vi "Find Color.vi"(8 "error in (no error)":errorcluster, 10 "Color Selected":u32(colorbox), 11 "ColorSelector in":refnum<class "ColorSelector.lvclass">) -> (0 "error out":errorcluster, 3 "ColorSelector out":refnum<class "ColorSelector.lvclass">)   [LabVIEW 2015, in "ColorSelector.lvclass"]
doc: "This VI finds the closest color in the Color Selector.\n<b> </b> <b> </b>\n©2017 Q Software Innovations, LLC (QSI)\nwritten by Quentin Alldredge\nproduced in LabVIEW 2015\n\nsupport@qsoftwareinnovations.com\nwww.qsoftwareinnovations.com\n\nAll rights reserved.\n\nRedistribution and use in source and binary forms, with or without modification, are permitted provided that the following conditions are met:\n\n * Redistributions of source code must retain the above copyright notice, this list of conditions and the following disclaimer.\n * Redistributions in binary form must reproduce the above copyright notice, this list of conditions and the following disclaimer in the documentation and/or other materials provided with the distribution.\n * Neither the name of Q Software Innovations, LLC. nor the names of its contributors may be used to endorse or promote products derived from this software without specific prior written permission.\n\nTHIS SOFTWARE IS PROVIDED BY THE COPYRIGHT HOLDERS AND CONTRIBUTORS \"AS IS\" AND ANY EXPRESS OR IMPLIED WARRANTIES, INCLUDING, BUT NOT LIMITED TO, THE IMPLIED WARRANTIES OF MERCHANTABILITY AND FITNESS FOR A PARTICULAR PURPOSE ARE DISCLAIMED. IN NO EVENT SHALL THE COPYRIGHT OWNER OR CONTRIBUTORS BE LIABLE FOR ANY DIRECT, INDIRECT, INCIDENTAL, SPECIAL, EXEMPLARY, OR CONSEQUENTIAL DAMAGES (INCLUDING, BUT NOT LIMITED TO, PROCUREMENT OF SUBSTITUTE GOODS OR SERVICES; LOSS OF USE, DATA, OR PROFITS; OR BUSINESS INTERRUPTION) HOWEVER CAUSED AND ON ANY THEORY OF LIABILITY, WHETHER IN CONTRACT, STRICT LIABILITY, OR TORT (INCLUDING NEGLIGENCE OR OTHERWISE) ARISING IN ANY WAY OUT OF THE USE OF THIS SOFTWARE, EVEN IF ADVISED OF THE POSSIBILITY OF SUCH DAMAGE."
uses:
  ColorSelector.lvclass
  <vilib>/Utility/miscctls.llb/LVPoint32TypeDef.ctl
  Read ColorSelectPic.vi
  Write ColorGridCoords.vi
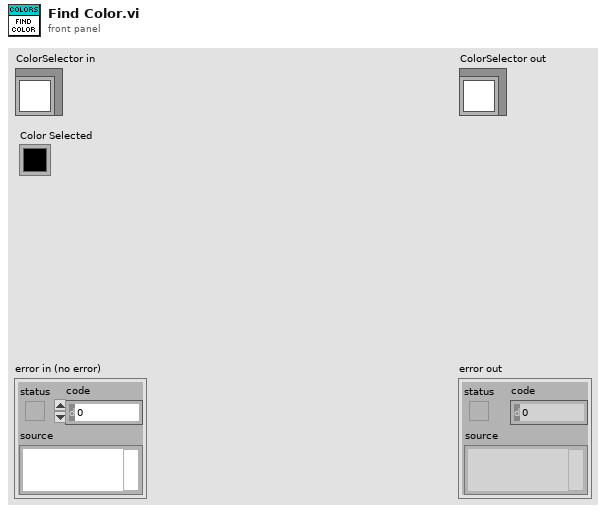
[diagram p1: front panel]
types:
  T1 = typedef "LVPoint32TypeDef.ctl" = cluster{"Horizontal":i32, "Vertical":i32}
  T2 = typedef "imagedata.ctl" = cluster{"image type":i32, "image depth":i32, "image":u8[], "mask":u8[], "colors":u32[], "Rectangle":cluster{"left":i16, "top":i16, "right":i16, "bottom":i16}}
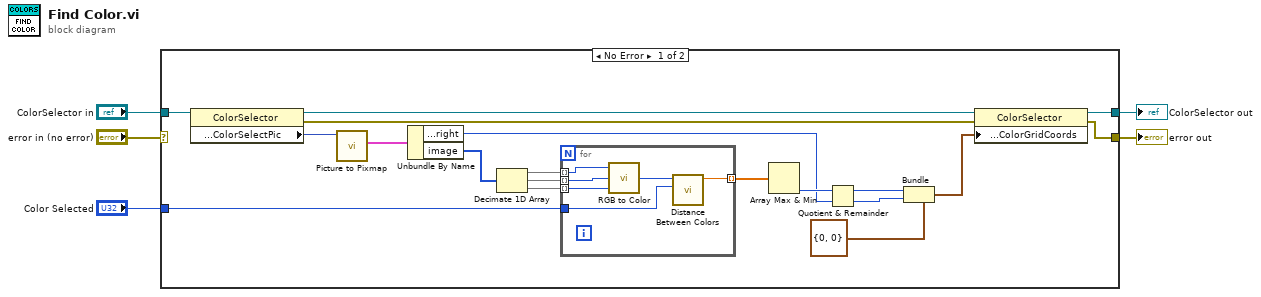
[diagram p0: block diagram]
diagram:
  n1 = case shown="No Error" "error in (no error)" {
    selector: "error in (no error)" -> [_ w32]
    tunnel: [w6 w32] -> w4
    tunnel: [w12 w31] -> w2
    tunnel: "ColorSelector in" -> [w24 w31]
    tunnel: "Color Selected" -> [w14 _]
    frame No Error {
      n2 = property class="ColorSelector"(reference=w24) -> (reference out=w23:refnum<class "ColorSelector.lvclass">, error out=w7:errorcluster, "State Data:Accessors:ColorSelectPic"=w22:picture)  [unwired: 1 in]
      n3 = call <vilib>:"Picture to Pixmap.vi"("picture"=w22) -> ("image data"=w21:T2)  [unwired: 9 in, 1 out]
      n4 = Unbundle By Name(w21) -> ("Rectangle.right"=w13:i16, "image"=w15:u8[])
      n5 = Decimate 1D Array(w15) -> (w16:u8[], w17:u8[], w18:u8[])
      n6 = for {
        tunnel: w16 -> [w28] mode=indexing
        tunnel: w17 -> [w29] mode=indexing
        tunnel: w18 -> [w30] mode=indexing
        tunnel: w14 -> [w26]
        tunnel: [w25] -> w19 mode=indexing
        n7 = call <vilib>:"RGB to Color.vi"("B"=w30, "G"=w29, "R"=w28) -> ("Color"=w27:u32)
        n8 = call "Distance Between Colors.vi"("Color 2"=w26, "Color 1"=w27) -> ("Distance"=w25:dbl)  [unwired: 8 in, 1 out]
      }
      n9 = Array Max & Min(array=w19) -> (min index (indices)=w20:i32)  [unwired: 3 out]
      n10 = Quotient & Remainder(x=w20, y=w13) -> (x-y*floor(x/y)=w10:i32, floor(x/y)=w9:i32)
      n11 = Bundle(cluster=T1 {"Horizontal"=0, "Vertical"=0} ("ColorGridCoords"), "Horizontal"=w10, "Vertical"=w9) -> (w8:T1)
      n12 = property class="ColorSelector"(reference=w23, error in=w7, "State Data:Accessors:ColorGridCoords"=w8) -> (reference out=w12:refnum<class "ColorSelector.lvclass">, error out=w6:errorcluster)
    }
    frame Error {
    }
  }
  "error out" <- w4
  "ColorSelector out" <- w2
